vi "Four Element Byte Array to U32.vi"(1 "Four Element Byte Array":u8[](array[numeric])) -> (0 "U32 out":u32)   [LabVIEW 2009]
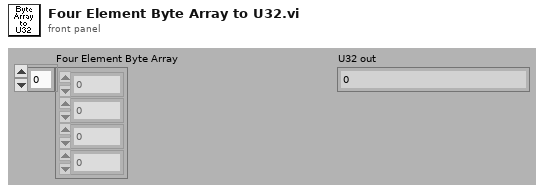
[diagram p1: front panel]
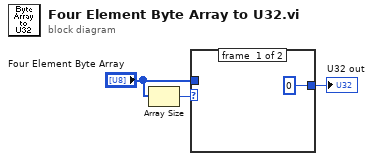
[diagram p0: block diagram]
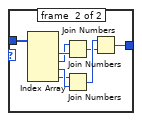
[diagram p2: hidden frame]
diagram:
  n1 = Array Size(array="Four Element Byte Array") -> (size(s)=w2:i32)
  n2 = case shown="4" w2 {
    tunnel: "Four Element Byte Array" -> [_ w12]
    tunnel: [u32 0 ("Numeric") w11] -> w1
    frame #0 {
    }
    frame #1 {
      n3 = Index Array(array=w12) -> (element #1=w10:u8, element #2=w9:u8, element #3=w8:u8, element #4=w7:u8)  [unwired: 4 in]
      n4 = Join Numbers(hi=w9, lo=w10) -> ((hi.lo)=w5:u16)
      n5 = Join Numbers(hi=w7, lo=w8) -> ((hi.lo)=w6:u16)
      n6 = Join Numbers(hi=w6, lo=w5) -> ((hi.lo)=w11:u32)
    }
  }
  "U32 out" <- w1
